vi "Create Class ObjectData DVR.vi"(8 "error in (no error)":errorcluster, 11 "Log_Engine in":refnum<class "Log_Engine.lvclass">) -> (0 "error out":errorcluster, 3 "Log_Engine out":refnum<class "Log_Engine.lvclass">)   [LabVIEW 2019, in "Log_Engine.lvclass"]
doc: "Developed by Kevin Thompson\nkevin@thompsonengineering.net\n\nCopyright 2018\nThompson Engineering, LLC"
uses:
  Log_Engine.lvclass
  DataTypes/ObjData--cluster.ctl
  DataTypes/Settings--cluster.ctl
  DataTypes/Public Events--cluster.ctl
  Common/DataTypes/TD Async CmdMsg EventData--cluster.ctl
  DataTypes/LogStateChg EvData--cluster.ctl
  DataTypes/LogStateEvData--cluster.ctl
  Common/DataTypes/LogState--enum.ctl
  DataTypes/TDMSStateChg EvData--cluster.ctl
  DataTypes/TDMSStateEvData--cluster.ctl
  Common/DataTypes/TDMSState--enum.ctl
  DataTypes/Dependency--cluster.ctl
  Config/Config.lvclass
  DAQ_Engine/DAQ_Engine.lvclass
  DataTypes/Read Data--cluster.ctl
  Common/DataTypes/InverterWaveforms--QRef.ctl
  Common/DataTypes/InverterWaveforms--cluster.ctl
  Common/DataTypes/ChannelWaveforms--cluster.ctl
  Log_Engine.lvclass/Log_Engine.ctl
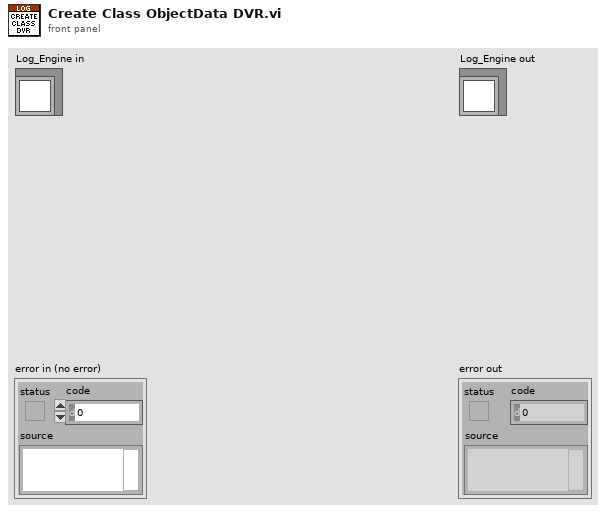
[diagram p1: front panel]
types:
  T1 = typedef "Log_Engine.lvclass/ObjData--cluster.ctl" = cluster{"Settings":T2, "Public Events":T3, "Dependency":T4, "ReadData-placeholder":T5, "VISA-placeholder":refnum<visa-resource-name>, "InverterWaveformsQ":T6, "LogState":T7, "TDMSState":T8}
  T2 = typedef "Log_Engine.lvclass/Settings--cluster.ctl" = cluster{"Simulation":bool, "TDMS_FolderPath":string, "CSV_FolderPath":string, "TDMS_FileName_Prefix":string, "CSV_FileName_Prefix":string, "TDMS_LogDuration(s)":dbl, "CSV_LogDuration(s)":dbl}
  T3 = typedef "Log_Engine.lvclass/Public Events--cluster.ctl" = cluster{"Log_Engine.AsyncCmd Event":refnum<user-event>, "Log_Engine.AsyncMsg Event":refnum<user-event>, "stop process":refnum<user-event>, "Log_Engine.LogStateChg Ev":refnum<user-event>, "Log_Engine.TDMSStateChg Ev":refnum<user-event>}
  T4 = typedef "Log_Engine.lvclass/Dependency--cluster.ctl" = cluster{"Config":refnum<class "Config.lvclass">, "DAQ_Engine":refnum<class "DAQ_Engine.lvclass">}
  T5 = typedef "Log_Engine.lvclass/Read Data--cluster.ctl" = cluster{"Data":dbl}
  T6 = typedef "InverterWaveforms--QRef.ctl" = refnum<queue>
  T7 = typedef "LogState--enum.ctl" = enum16{"Unknown", "Stopped", "Running", "Error"}
  T8 = typedef "TDMSState--enum.ctl" = enum16{"Unknown", "Stopped", "Running", "Error"}
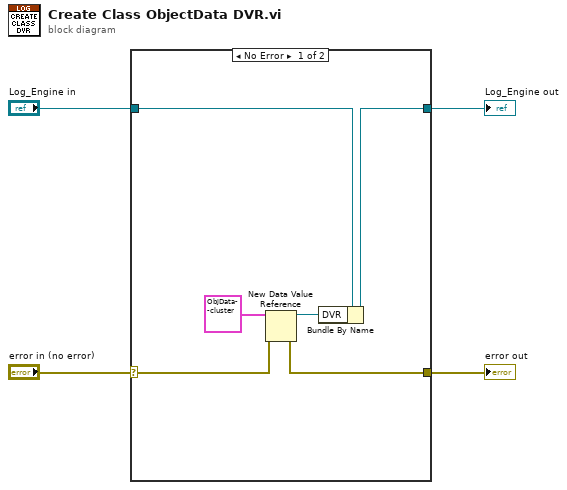
[diagram p0: block diagram]
diagram:
  n1 = case shown="No Error" "error in (no error)" {
    selector: "error in (no error)" -> [w9 w12]
    tunnel: [w8 w12] -> w3
    tunnel: [w6 w11] -> w1
    tunnel: "Log_Engine in" -> [w7 w11]
    frame No Error {
      n2 = New Data Value Reference(data value=T1 {"Settings"={"Simulation"=FALSE, "TDMS_FolderPath"="", "CSV_FolderPath"="", "TDMS_FileName_Prefix"="", "CSV_FileName_Prefix"="", "TDMS_LogDuration(s)"=0.0, "CSV_LogDuration(s)"=0.0}, "Public Events"={"Log_Engine.AsyncCmd Event"=refnum, "Log_Engine.AsyncMsg Event"=refnum, "stop process"=refnum, "Log_Engine.LogStateChg Ev"=refnum, "Log_Engine.TDMSStateChg Ev"=refnum}, "Dependency"={"Config"=refnum, "DAQ_Engine"=refnum}, "ReadData-placeholder"={"Data"=0.0}, "VISA-placeholder"="", "InverterWaveformsQ"=refnum, "LogState"=enum."Unknown", "TDMSState"=enum."Unknown"} ("ObjData"), error in=w9) -> (data value reference=w10:refnum<data-value>, error out=w8:errorcluster)
      n3 = Bundle By Name(cluster=w7, "DVR"=w10) -> (w6:refnum<class "Log_Engine.lvclass">)
    }
    frame Error {
    }
  }
  "error out" <- w3
  "Log_Engine out" <- w1
